vi "Get Todo Bookmarks.vi"(6 "open VI references? (False)":bool, 8 "error in (no error)":errorcluster, 11 "Directory to Search":path) -> (0 "error out":errorcluster, 2 "todo bookmarks":map{path, T1}(c390))   [LabVIEW 2020]
uses:
  <vilib>/Utility/miscctls.llb/LVBookmarkInfoTypeDef.ctl
  af485d53-b5a2-4225-9b29-f30f09fd7990.vi
panel:
  out "Errors":path[](array[path])
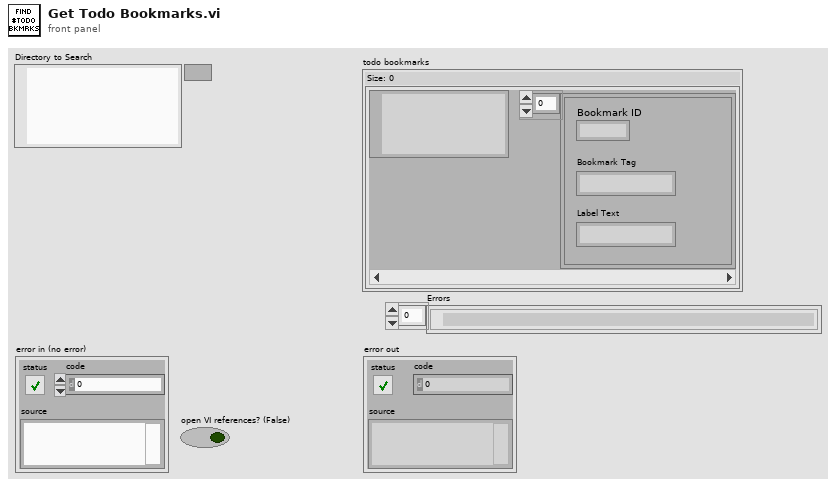
[diagram p1: front panel]
types:
  T1 = typedef "LVBookmarkInfoTypeDef.ctl" = cluster{"Bookmark ID":u32, "Bookmark Tag":string, "Label Text":string}[]
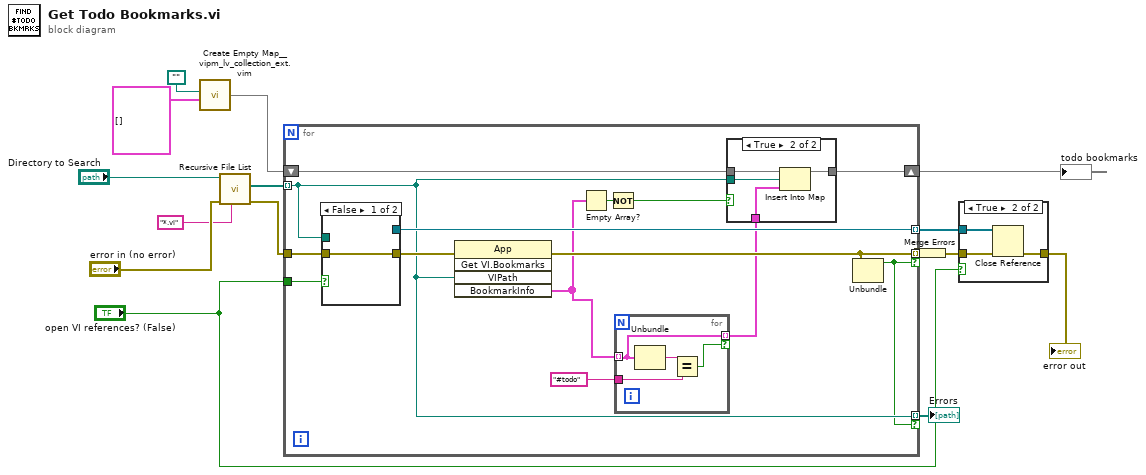
[diagram p0: block diagram]
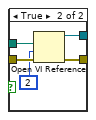
[diagram p3: hidden frame]
diagram:
  n1 = call "Create Empty Map__vipm_lv_collection_ext.vim"("value type"=T1 [] ("Bookmark Information"), "key type"=path "" ("VI Path")) -> ("empty map"=w10:map{path, T1})  [unwired: 8 in]
  n2 = call <vilib>:"Recursive File List.vi"("pattern"="*.vi", "error in (no error)"="error in (no error)", "Folder Path"="Directory to Search") -> ("error out"=w13:errorcluster, "All Files in Dir"=w5:path[])  [unwired: 4 in, 3 out]
  n3 = for {
    tunnel: w5 -> [w17] mode=indexing
    tunnel: [w28] -> w6 mode=indexing
    shift-right: [w26] -> w15
    shift-left: w10 -> [w21]
    tunnel: w13 -> [w27]
    tunnel: [w24] -> w7 mode=indexing if=w16
    tunnel: "open VI references? (False)" -> [w18]
    tunnel: [w17] -> w1 mode=indexing if=w16
    n4 = case shown="False" w18 {
      tunnel: [w30 w35] -> w29
      tunnel: [_ w34] -> w28
      tunnel: w27 -> [w30 w33]
      tunnel: w17 -> [_ w31]
      frame False {
      }
      frame True {
        n5 = Open VI Reference(vi path=w31, options=2, error in (no error)=w33) -> (vi reference=w34:refnum<vi>, error out=w35:errorcluster)  [unwired: 3 in]
      }
    }
    n6 = invoke class="App" method="Get VI.Bookmarks"(error in=w29, "VIPath"=w17) -> (error out=w24:errorcluster, "BookmarkInfo"=w20:T1)  [unwired: 3 in, 3 out]
    n7 = Empty Array?(array=w20) -> (empty?=w25:bool)
    n8 = Not(x=w25) -> (.not. x?=w23:bool)
    n9 = for {
      tunnel: w20 -> [w37] mode=indexing
      tunnel: "#todo" ("Bookmark Tag") -> [w38]
      tunnel: [w37] -> w19 mode=indexing if=w36
      n10 = Unbundle(w37) -> ("Bookmark Tag"=w39:string)  [unwired: 2 out]
      n11 = Equal?(x=w39, y=w38) -> (x = y?=w36:bool)
    }
    n12 = case shown="True" w23 {
      tunnel: w21 -> [w40 w44]
      tunnel: [w40 w43] -> w26
      tunnel: w17 -> [_ w42]
      tunnel: w19 -> [_ w41]
      frame False {
      }
      frame True {
        n13 = Insert Into Map(map in=w44, key=w42, value=w41) -> (map out=w43:map{path, T1})  [unwired: 2 out]
      }
    }
    n14 = Unbundle(w24) -> ("status"=w16:bool)  [unwired: 2 out]
  }
  "todo bookmarks" <- w15
  "Errors" <- w1
  n15 = Merge Errors(w7) -> (w12:errorcluster)
  n16 = case shown="True" "open VI references? (False)" {
    tunnel: w12 -> [w45 w48]
    tunnel: [w45 w47] -> w11
    tunnel: w6 -> [_ w46]
    frame False {
    }
    frame True {
      n17 = Close Reference(reference=w46, error in (no error)=w48) -> (error out=w47:errorcluster)
    }
  }
  "error out" <- w11
